vi "TekAFG3102_userEvent.vi"() -> ()   [LabVIEW 2015]
uses:
  VIstatus.ctl
  NetworkStream/NetworkStreamReceiverStatusEventCluster.ctl
  NetworkStream/NetworkStream.lvlib
panel:
  out "division result":dbl
  in  "Numeric":dbl
  in  "upadate variable":bool
  in  "Stop program":bool
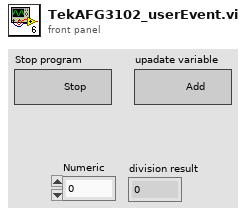
[diagram p1: front panel]
types:
  T1 = typedef "VIstatus.ctl" = enum16{"initializing", "running", "exiting"}
  T2 = typedef "NetworkStream.lvlib/NetworkStreamReceiverStatusEventCluster.ctl" = cluster{"Status":string, "Data":variant, "SequenceNumber":u64}
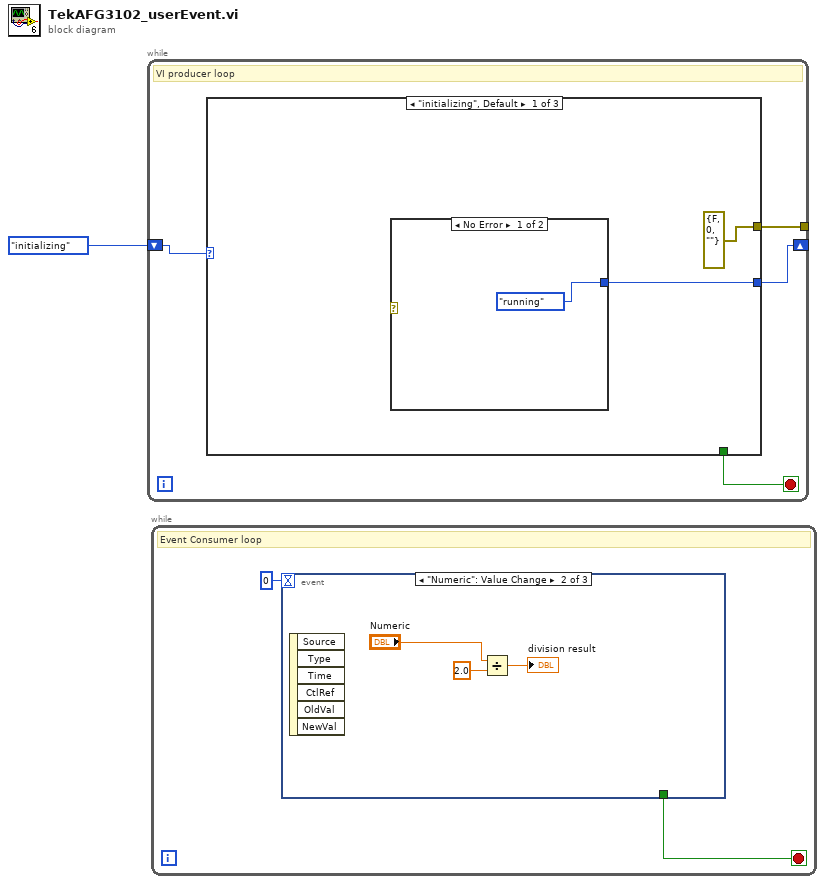
[diagram p0: block diagram]
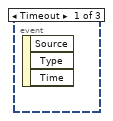
[diagram p2: hidden frame]
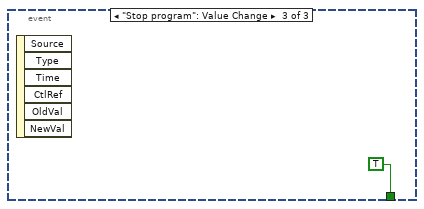
[diagram p3: hidden frame]
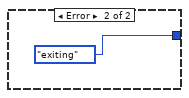
[diagram p4: hidden frame]
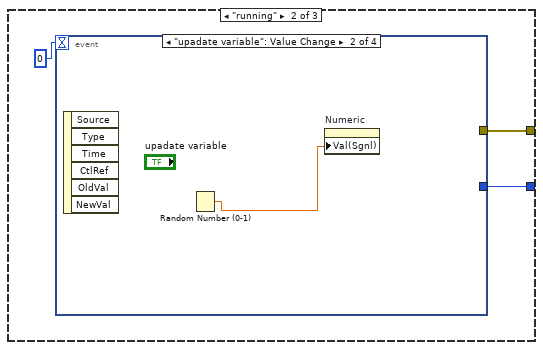
[diagram p5: hidden frame]
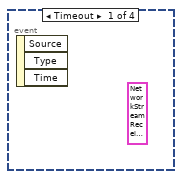
[diagram p6: hidden frame]
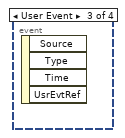
[diagram p7: hidden frame]
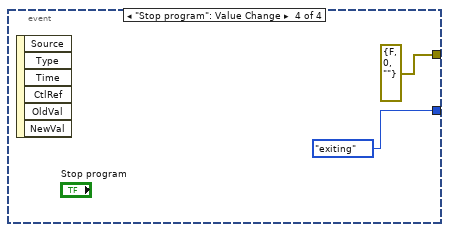
[diagram p8: hidden frame]
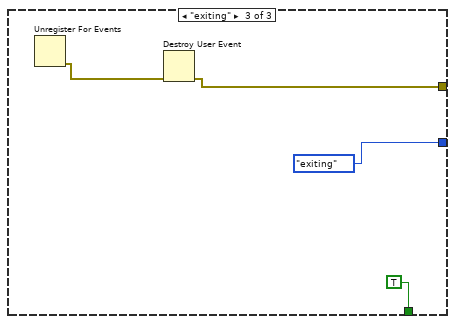
[diagram p9: hidden frame]
diagram:
  n1 = while {
    tunnel: [w4] -> _
    shift-right: [w3] -> _
    shift-left: VIstatus."initializing" ("DeviceState") -> [w5]
    stop <- w2 stop-if-true
    # "VI producer loop"
    n2 = case shown="\"initializing\", Default" w5 {
      tunnel: [errorcluster {"status"=FALSE, "code"=0, "source"=""} ("error out") w11 w17] -> w4
      tunnel: [w6 w10 VIstatus."exiting" ("DeviceState")] -> w3
      tunnel: [_ _ TRUE] -> w2
      frame "initializing", Default {
        n3 = case shown="No Error" {
          selector: _ -> [_ _]
          tunnel: [VIstatus."running" ("DeviceState") VIstatus."exiting" ("DeviceState")] -> w6
          frame No Error {
          }
          frame Error {
          }
        }
      }
      frame "running" {
        n4 = event shown="[1] \"upadate variable\": Value Change" {
          selector: _ -> [_ _ _ _]
          dyn-events: _ -> [_ _ _ _]
          timeout: 0 -> [_ _ _ _]
          tunnel: [_ _ _ errorcluster {"status"=FALSE, "code"=0, "source"=""} ("error out")] -> w11
          tunnel: [_ _ _ VIstatus."exiting" ("DeviceState")] -> w10
          event Timeout {
            (unwired) T2 {"Status"="", "Data"=variant, "SequenceNumber"=0} ("event data")
            n5 = event-data() -> ()  [unwired: 1 in, 3 out]
          }
          event "upadate variable": Value Change {
            n6 = event-data() -> ()  [unwired: 1 in, 6 out]
            n7 = Random Number (0-1)() -> (number: 0 to 1=w13:dbl)
            n8 = property on="Numeric" class="DigNum (strict)"("Val(Sgnl)"=w13) -> ()  [unwired: 2 in, 2 out]
          }
          event User Event {
            n9 = event-data() -> ()  [unwired: 1 in, 4 out]
          }
          event "Stop program": Value Change {
            n10 = event-data() -> ()  [unwired: 1 in, 6 out]
          }
        }
      }
      frame "exiting" {
        n11 = Unregister For Events() -> (error out=w18:errorcluster)  [unwired: 2 in]
        n12 = Destroy User Event(error in=w18) -> (error out=w17:errorcluster)  [unwired: 1 in]
      }
    }
  }
  n13 = while {
    stop <- w21 stop-if-true
    # "Event Consumer loop"
    n14 = event shown="[1] \"Numeric\": Value Change" {
      selector: _ -> [_ _ _]
      dyn-events: _ -> [_ _ _]
      timeout: 0 -> [_ _ _]
      tunnel: [_ _ TRUE] -> w21
      event Timeout {
        n15 = event-data() -> ()  [unwired: 1 in, 3 out]
      }
      event "Numeric": Value Change {
        n16 = event-data() -> ()  [unwired: 1 in, 6 out]
        n17 = Divide(x="Numeric", y=2.0) -> (x/y=→"division result":dbl)
      }
      event "Stop program": Value Change {
        n18 = event-data() -> ()  [unwired: 1 in, 6 out]
      }
    }
  }
